vi "Maestro principal.vi"() -> ()   [LabVIEW 2012]
doc: "Use this template to build a standard state machine design pattern. Each state executes code and determines which state to transition to. Contrast this design pattern with the User Interface Event Handler pattern, in which code executes in response to user actions. Contrast this design pattern also with the Queued Message Handler pattern, in which each message handling code can queue zero or more new messages.\nNote: This template does not contain the most recent programming guidelines recommended by National Instruments. For a complete, project-based implementation of the Standard State Machine pattern, use the Create Project dialog box instead of this template."
uses:
  Estados.ctl
  Global Variables.vi
  Extractor Matrices.vi
panel:
  in  "Obtener patrones":bool
  out "Array  Target 0":i32[](array[numeric])
  out "Array  Target A":i32[](array[numeric])
  out "Path Rlativo":path
  out "Numeric":i32
  out "StackFotos":string[](array[string])
  out "Letras":string
  out "Numeros":string
  in  "Next Image":bool
  out "Array  SAT":u8[](array[numeric])
  out "Array  VAL":u8[](array[numeric])
  out "Array  BLUE":u8[](array[numeric])
  out "Array GREEN":u8[](array[numeric])
  out "Array RED":u8[](array[numeric])
  in  "Salir":bool
  in  "Clear ROI":bool
  in  "OK ROI":bool
  in  "Cancel":bool
  in  "OK":bool
  in  "Path":path
  out "Original":T1(plugin-control)
  in  "Load Button":bool
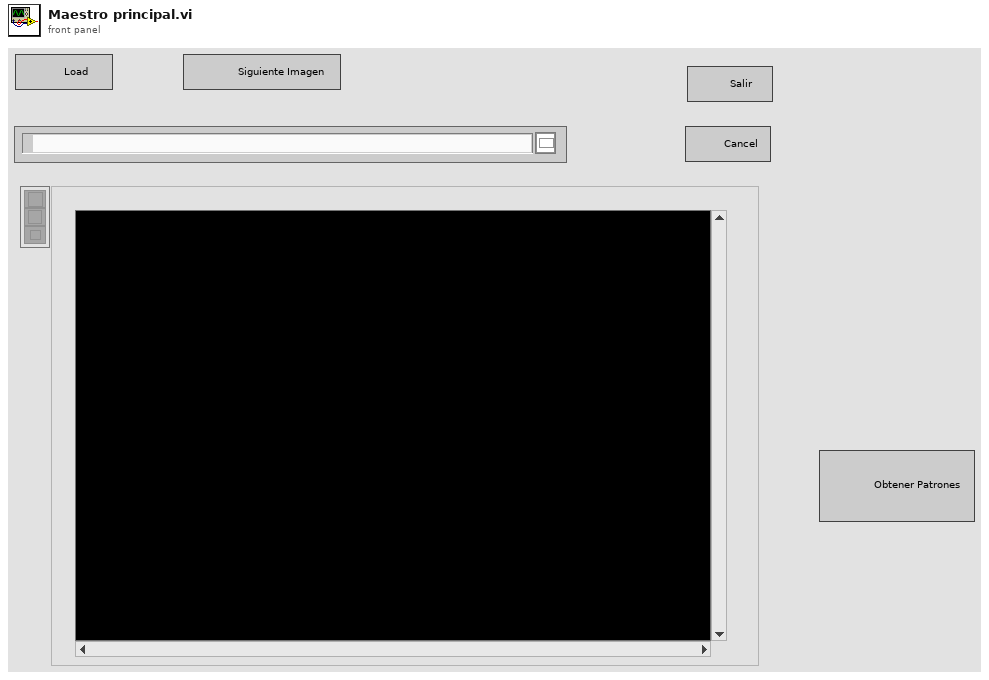
[diagram p1: front panel]
types:
  T1 = typedef "IMAQ Image.ctl" = refnum<image>
  T2 = typedef "Estados.ctl" = enum16{"Initialize", "Stop", "Load", "Next Image", "Get Planes", "Get pixels", "Save"}
  T3 = typedef "Image Type" = u32
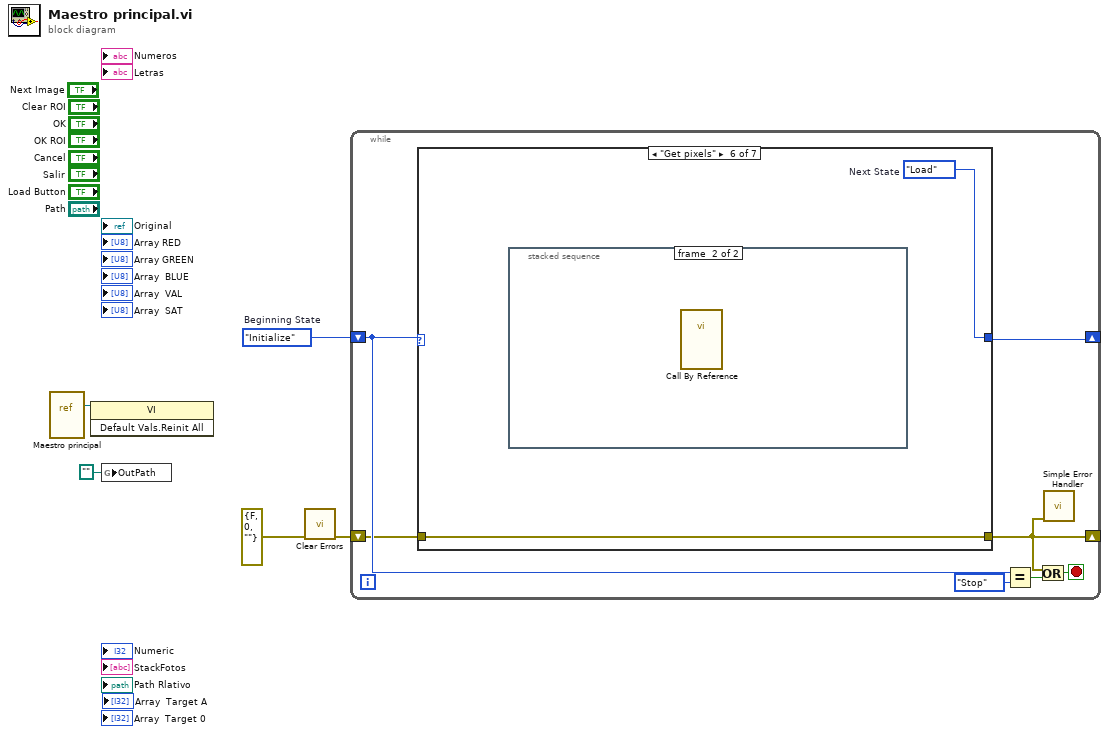
[diagram p0: block diagram]
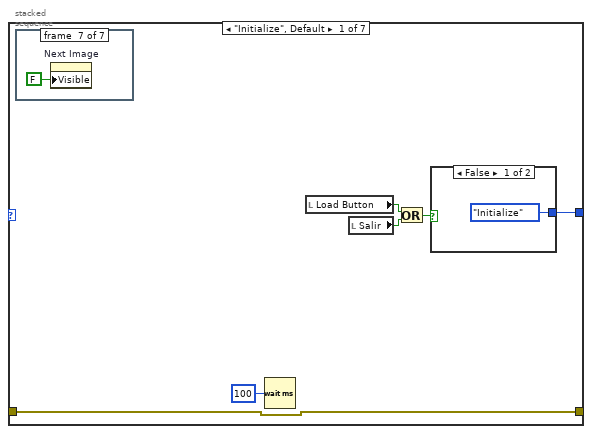
[diagram p2: hidden frame]
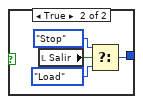
[diagram p3: hidden frame]
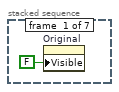
[diagram p4: hidden frame]
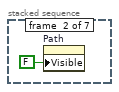
[diagram p5: hidden frame]
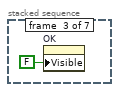
[diagram p6: hidden frame]
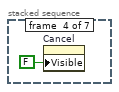
[diagram p7: hidden frame]
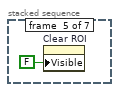
[diagram p8: hidden frame]
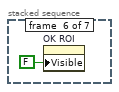
[diagram p9: hidden frame]
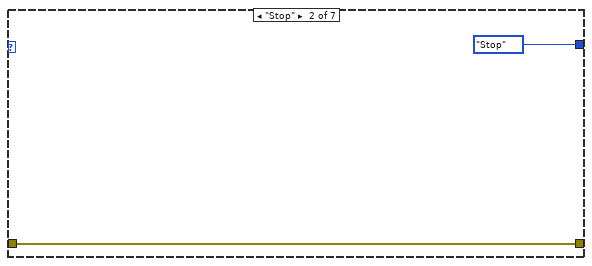
[diagram p10: hidden frame]
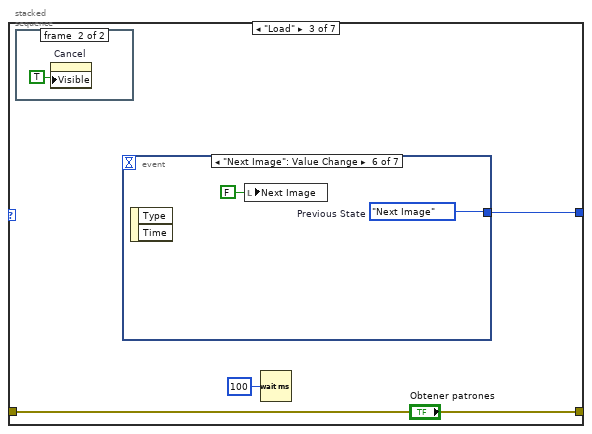
[diagram p11: hidden frame]
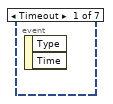
[diagram p12: hidden frame]
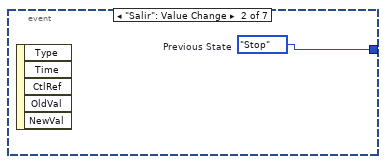
[diagram p13: hidden frame]
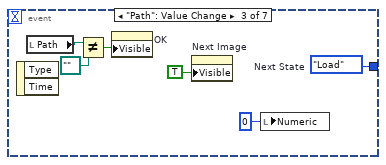
[diagram p14: hidden frame]
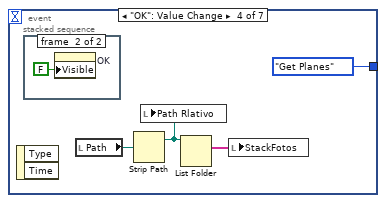
[diagram p15: hidden frame]
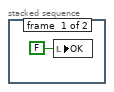
[diagram p16: hidden frame]
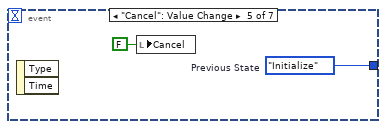
[diagram p17: hidden frame]
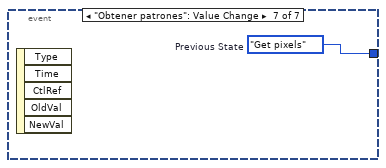
[diagram p18: hidden frame]
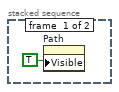
[diagram p19: hidden frame]
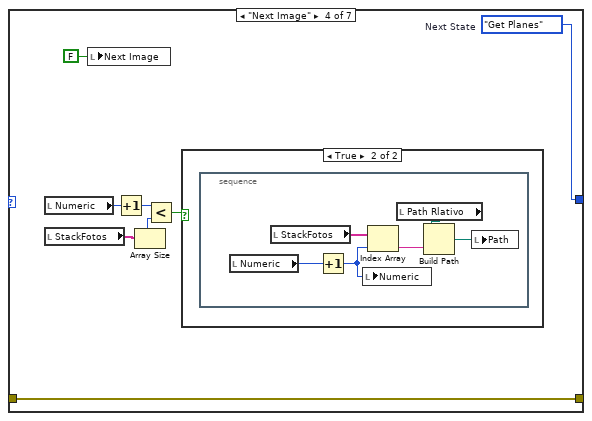
[diagram p20: hidden frame]
diagram:
  w5 = Estados."Initialize"  # Beginning State
  n1 = vi-ref "Maestro principal.vi"() -> (w4:refnum<vi>)
  n2 = invoke class="VI" method="Default Vals.Reinit All"(reference=w4) -> ()  [unwired: 2 in, 3 out]
  n3 = global write "Global Variables.vi" "OutPath"(path "") -> ()
  n4 = call <vilib>:"Clear Errors.vi"("error in (no error)"=errorcluster {"status"=FALSE, "code"=0, "source"=""}) -> ("error out"=w3:errorcluster)  [unwired: 6 in]
  n5 = while {
    shift-right: [w10] -> _
    shift-left: w5 -> [w11]
    shift-right: [w6] -> _
    shift-left: w3 -> [w9]
    stop <- w7 stop-if-true
    n6 = case shown="\"Get pixels\"" w11 {
      tunnel: [w13 Estados."Stop" ("Next State") w34 w63 w78 w81 Estados."Save" ("States")] -> w10
      tunnel: w9 -> [w17 w31 w33 w62 w77 w82 w89]
      tunnel: [w17 w31 w33 w62 w77 w82 w89] -> w6
      frame "Initialize", Default {
        n7 = stacked-sequence {
          frame #0 {
            n8 = property on="Original" class="ImageControl"("Visible"=FALSE) -> ()  [unwired: 2 in, 2 out]
          }
          frame #1 {
            n9 = property on="Path" class="Path"("Visible"=FALSE) -> ()  [unwired: 2 in, 2 out]
          }
          frame #2 {
            n10 = property on="OK" class="Bool (strict)"("Visible"=FALSE) -> ()  [unwired: 2 in, 2 out]
          }
          frame #3 {
            n11 = property on="Cancel" class="Bool (strict)"("Visible"=FALSE) -> ()  [unwired: 2 in, 2 out]
          }
          frame #4 {
            n12 = property on="Clear ROI" class="Bool (strict)"("Visible"=FALSE) -> ()  [unwired: 2 in, 2 out]
          }
          frame #5 {
            n13 = property on="OK ROI" class="Bool (strict)"("Visible"=FALSE) -> ()  [unwired: 2 in, 2 out]
          }
          frame #6 {
            n14 = property on="Next Image" class="Bool (strict)"("Visible"=FALSE) -> ()  [unwired: 2 in, 2 out]
          }
        }
        n15 = Wait (ms)(milliseconds to wait=u32 100) -> ()  [unwired: 1 out]
        n16 = local read "Load Button"() -> (w16:bool)
        n17 = local read "Salir"() -> (w15:bool)
        n18 = Or(x=w16, y=w15) -> (x .or. y?=w14:bool)
        n19 = case shown="False" w14 {
          tunnel: [Estados."Initialize" w20] -> w13
          frame False {
          }
          frame True {
            n20 = local read "Salir"() -> (w23:bool)
            n21 = Select(t=Estados."Stop", s=w23, f=Estados."Load") -> (s? t:f=w20:T2)
          }
        }
      }
      frame "Stop" {
      }
      frame "Load" {
        n22 = stacked-sequence {
          frame #0 {
            n23 = property on="Path" class="Path"("Visible"=TRUE) -> ()  [unwired: 2 in, 2 out]
          }
          frame #1 {
            n24 = property on="Cancel" class="Bool (strict)"("Visible"=TRUE) -> ()  [unwired: 2 in, 2 out]
          }
        }
        n25 = event shown="[5] \"Next Image\": Value Change" {
          selector: _ -> [_ _ _ _ _ _ _]
          dyn-events: _ -> [_ _ _ _ _ _ _]
          timeout: _ -> [_ _ _ _ _ _ _]
          tunnel: [_ w36 w39 Estados."Get Planes" w50 w52 w53] -> w34
          event Timeout {
            n26 = event-data() -> ()  [unwired: 1 in, 2 out]
          }
          event "Salir": Value Change {
            w36 = Estados."Stop"  # Previous State
            n27 = event-data() -> ()  [unwired: 1 in, 5 out]
          }
          event "Path": Value Change {
            w39 = Estados."Load"  # Next State
            n28 = event-data() -> ()  [unwired: 1 in, 2 out]
            n29 = local read "Path"() -> (w42:path)
            n30 = Not Equal?(x=w42, y=path "") -> (x != y?=w41:bool)
            n31 = property on="OK" class="Bool (strict)"("Visible"=w41) -> ()  [unwired: 2 in, 2 out]
            n32 = property on="Next Image" class="Bool (strict)"("Visible"=TRUE) -> ()  [unwired: 2 in, 2 out]
            n33 = local write "Numeric"(0 ("Numeric")) -> ()
          }
          event "OK": Value Change {
            n34 = event-data() -> ()  [unwired: 1 in, 2 out]
            n35 = stacked-sequence {
              frame #0 {
                n36 = local write "OK"(FALSE ("OK")) -> ()
              }
              frame #1 {
                n37 = property on="OK" class="Bool (strict)"("Visible"=FALSE) -> ()  [unwired: 2 in, 2 out]
              }
            }
            n38 = local read "Path"() -> (w44:path)
            n39 = Strip Path(path=w44) -> (stripped path=w45:path)  [unwired: 1 out]
            n40 = local write "Path Rlativo"(w45) -> ()
            n41 = List Folder(path=w45) -> (filenames=w43:string[])  [unwired: 3 in, 3 out]
            n42 = local write "StackFotos"(w43) -> ()
          }
          event "Cancel": Value Change {
            w50 = Estados."Initialize"  # Previous State
            n43 = event-data() -> ()  [unwired: 1 in, 2 out]
            n44 = local write "Cancel"(FALSE ("Cancel")) -> ()
          }
          event "Next Image": Value Change {
            w52 = Estados."Next Image"  # Previous State
            n45 = event-data() -> ()  [unwired: 1 in, 2 out]
            n46 = local write "Next Image"(FALSE ("Next Image")) -> ()
          }
          event "Obtener patrones": Value Change {
            w53 = Estados."Get pixels"  # Previous State
            n47 = event-data() -> ()  [unwired: 1 in, 5 out]
          }
        }
        n48 = Wait (ms)(milliseconds to wait=u32 100) -> ()  [unwired: 1 out]
      }
      frame "Next Image" {
        w63 = Estados."Get Planes"  # Next State
        n49 = local read "Numeric"() -> (w58:i32)
        n50 = local read "StackFotos"() -> (w61:string[])
        n51 = local write "Next Image"(FALSE ("Next Image")) -> ()
        n52 = Increment(x=w58) -> (x+1=w57:i32)
        n53 = Array Size(array=w61) -> (size(s)=w59:i32)
        n54 = Less?(x=w57, y=w59) -> (x < y?=w60:bool)
        n55 = case shown="True" w60 {
          frame False {
            n56 = One Button Dialog(message="Barrido de imágenes\ncompleto") -> ()  [unwired: 1 in, 1 out]
          }
          frame True {
            n57 = stacked-sequence {
              frame #0 {
                n58 = local read "Numeric"() -> (w70:i32)
                n59 = local read "StackFotos"() -> (w69:string[])
                n60 = Increment(x=w70) -> (x+1=w68:i32)
                n61 = local write "Numeric"(w68) -> ()
                n62 = Index Array(array=w69, index=w68) -> (element=w66:string)
                n63 = local read "Path Rlativo"() -> (w67:path)
                n64 = Build Path(base path=w67, name or relative path=w66) -> (appended path=w65:path)
                n65 = local write "Path"(w65) -> ()
              }
            }
          }
        }
      }
      frame "Get Planes" {
        w73 = T3 4 items=["Grayscale (U8)", "Grayscale (I16)", "Grayscale (SGL)", "Complex (CSG)", "RGB (U32)", "HSL (U32)", "RGB (U64)", "Grayscale (U16)"] ("Image Type")
        w78 = Estados."Load"  # Next State
        n66 = stacked-sequence {
          frame #0 {
            n67 = property on="Original" class="ImageControl"("Visible"=TRUE) -> ()  [unwired: 2 in, 2 out]
          }
        }
        n68 = Wait (ms)(milliseconds to wait=u32 100) -> ()  [unwired: 1 out]
        n69 = call "IMAQ Create"("Image Name"="Original", "Image Type"=w73) -> ("New Image"=w74:T1, "error out"=w75:errorcluster)  [unwired: 3 in]
        n70 = local read "Path"() -> (w72:path)
        n71 = call "IMAQ ReadFile"("File Path"=w72, "error in (no error)"=w75, "Image"=w74) -> ("Image Out"=w71:T1)  [unwired: 4 in, 4 out]
        n72 = local write "Original"(w71) -> ()
        n73 = global write "Global Variables.vi" "Image"(w71) -> ()
      }
      frame "Get pixels" {
        w81 = Estados."Load"  # Next State
        n74 = stacked-sequence {
          frame #0 {
            n75 = global read "Global Variables.vi" "OutPath"() -> (w85:path)
            n76 = Equal?(x=w85, y=path "") -> (x = y?=w83:bool)
            n77 = case shown="False" w83 {
              frame False {
              }
              frame True {
                n78 = stacked-sequence {
                  frame #0 {
                    n79 = One Button Dialog(message="Seleccione folder de salida") -> ()  [unwired: 1 in, 1 out]
                  }
                  frame #1 {
                    n80 = call <vilib>:"Application Directory.vi"() -> ("Application Directory"=w88:path)
                    n81 = call "File Dialog"("start path"=w88) -> ("selected path"=w87:path)  [unwired: 11 in, 3 out]
                    n82 = global write "Global Variables.vi" "OutPath"(w87) -> ()
                  }
                }
              }
            }
          }
          frame #1 {
            n83 = call-by-ref "?"() -> ()  [unwired: 14 in, 2 out]
          }
        }
      }
      frame "Save" {
      }
    }
    n84 = Equal?(x=w11, y=Estados."Stop" ("States")) -> (x = y?=w8:bool)
    n85 = Or(x=w6, y=w8) -> (x .or. y?=w7:bool)
    n86 = call <vilib>:"Simple Error Handler.vi"("error in (no error)"=w6) -> ()  [unwired: 4 in, 5 out]
  }
